vi "Get flattened data.vi"(8 "error in (no error)":errorcluster, 11 "U8 D Element in":refnum<class "U8 D Element.lvclass">) -> (0 "error out":errorcluster, 2 "Flattened data":u8[](array[numeric]), 3 "U8 D Element out":refnum<class "U8 D Element.lvclass">)   [LabVIEW 2018, in "D Datagrid Library.lvlib" / "U8 D Element.lvclass"]
uses:
  U8 D Element.lvclass
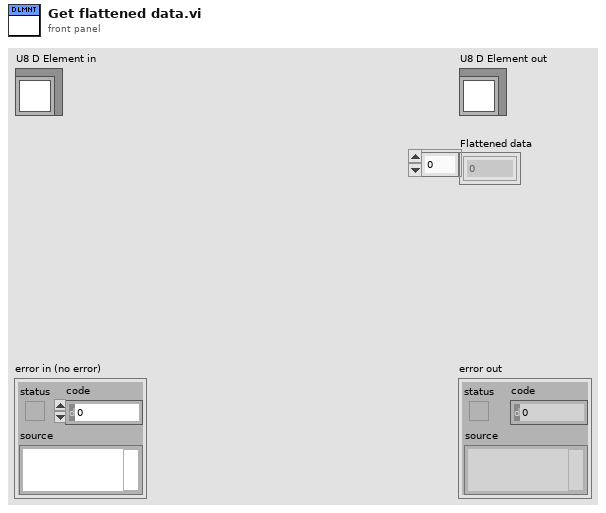
[diagram p1: front panel]
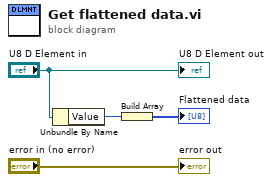
[diagram p0: block diagram]
diagram:
  n1 = Unbundle By Name("U8 D Element in") -> ("Value"=w2:u8)
  n2 = Build Array(w2) -> (→"Flattened data":u8[])
  "error out" <- "error in (no error)"
  "U8 D Element out" <- "U8 D Element in"
